vi "AG Quiz Page.vi"() -> ()   [LabVIEW 2012]
uses:
  Controls/Quiz Question.ctl
  Controls/StoredQuizAnswer.ctl
  Controls/Solution Type enum.ctl
  Controls/Problem Type enum.ctl
  Controls/Quiz Set Up.ctl
panel:
  in  "Previous 2":bool
  out "Student Answers":string[](array[string])
  in  "Resources":path[](array[path])
  in  "Previous":bool
  in  "Next":bool
  in  "Quiz Scrollbar":i32(c297)
  in  "Problem3":T1={"ProblemNum"=0, "Problem Type"={"Text"="", "Image"=bytes[0], "Text&Image"={"Text (&Image)"="", "Image (&text)"=bytes[0]}}, "Solution Type"={"Short Answer"="", "True/False"=enum."True", "Radio"=enum."E", "Multi"={"Numeric"=0.0, "String"="", "A"=FALSE, "B"=FALSE, "C"=FALSE, "D"=FALSE, "E"=TRUE}}, "Answer Color"=0, "Submit"=FALSE}
  in  "Problem2":T1={"ProblemNum"=0, "Problem Type"={"Text"="", "Image"=bytes[0], "Text&Image"={"Text (&Image)"="", "Image (&text)"=bytes[0]}}, "Solution Type"={"Short Answer"="", "True/False"=enum."True", "Radio"=enum."E", "Multi"={"Numeric"=0.0, "String"="", "A"=FALSE, "B"=FALSE, "C"=FALSE, "D"=FALSE, "E"=TRUE}}, "Answer Color"=0, "Submit"=FALSE}
  in  "Problem1":T1={"ProblemNum"=0, "Problem Type"={"Text"="", "Image"=bytes[0], "Text&Image"={"Text (&Image)"="", "Image (&text)"=bytes[0]}}, "Solution Type"={"Short Answer"="", "True/False"=enum."True", "Radio"=enum."E", "Multi"={"Numeric"=0.0, "String"="", "A"=FALSE, "B"=FALSE, "C"=FALSE, "D"=FALSE, "E"=TRUE}}, "Answer Color"=0, "Submit"=FALSE}
  in  "Problem0":T1={"ProblemNum"=0, "Problem Type"={"Text"="", "Image"=bytes[0], "Text&Image"={"Text (&Image)"="", "Image (&text)"=bytes[0]}}, "Solution Type"={"Short Answer"="", "True/False"=enum."True", "Radio"=enum."E", "Multi"={"Numeric"=0.0, "String"="", "A"=FALSE, "B"=FALSE, "C"=FALSE, "D"=FALSE, "E"=TRUE}}, "Answer Color"=0, "Submit"=FALSE}
  out "Quiz Set up Array":T2[](array[typedef])=[{"Text"="", "Problem Type"=enum."Text", "Solution Type"=enum."Text", "NumSolMin"=0.0, "NumSolMax"=0.0, "NumSolSigFig"=0, "StoreAnswer"=variant, "Picture"=bytes[0], "T/F_Solution"=FALSE, "ExactMatch"=FALSE, "TextAnswer"="", "MultiAnswer"={"MultiDescArray"=[], "MultiBoolArray"=[]}, "SigFig?"=FALSE}, {"Text"="", "Problem Type"=enum."Text", "Solution Type"=enum."Text", "NumSolMin"=0.0, "NumSolMax"=0.0, "NumSolSigFig"=0, "StoreAnswer"=variant, "Picture"=bytes[0], "T/F_Solution"=FALSE, "ExactMatch"=FALSE, "TextAnswer"="", "MultiAnswer"={"MultiDescArray"=[], "MultiBoolArray"=[]}, "SigFig?"=FALSE}, {"Text"="", "Problem Type"=enum."Text", "Solution Type"=enum."Text", "NumSolMin"=0.0, "NumSolMax"=0.0, "NumSolSigFig"=0, "StoreAnswer"=variant, "Picture"=bytes[0], "T/F_Solution"=FALSE, "ExactMatch"=FALSE, "TextAnswer"="", "MultiAnswer"={"MultiDescArray"=[], "MultiBoolArray"=[]}, "SigFig?"=FALSE}, {"Text"="", "Problem Type"=enum."Text", "Solution Type"=enum."Text", "NumSolMin"=0.0, "NumSolMax"=0.0, "NumSolSigFig"=0, "StoreAnswer"=variant, "Picture"=bytes[0], "T/F_Solution"=FALSE, "ExactMatch"=FALSE, "TextAnswer"="", "MultiAnswer"={"MultiDescArray"=[], "MultiBoolArray"=[]}, "SigFig?"=FALSE}]
  in  "stop":bool
  # "C:\\Users\\NIK12\\Desktop\\AG Quiz Image - Art.png"
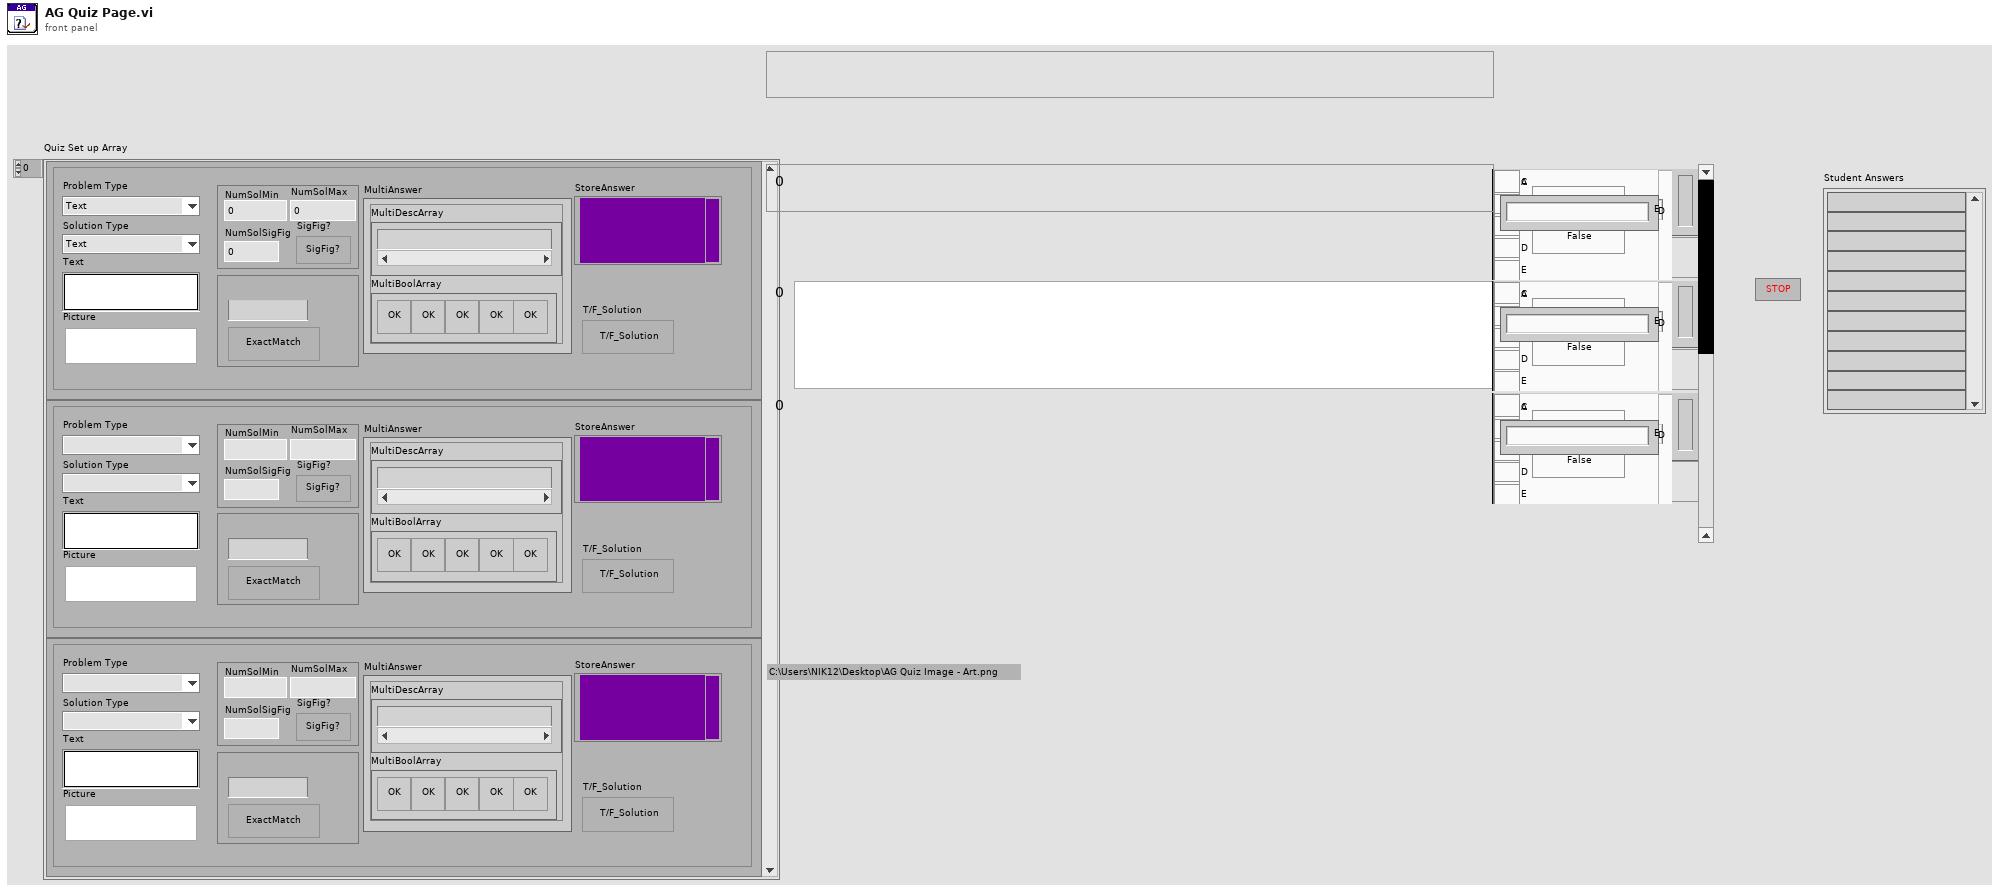
[diagram p1: front panel]
types:
  T1 = typedef "Quiz Question.ctl" = cluster{"ProblemNum":i32, "Problem Type":cluster{"Text":string, "Image":picture, "Text&Image":cluster{"Text (&Image)":string, "Image (&text)":picture}}, "Solution Type":cluster{"Short Answer":string, "True/False":enum32{"No Selection", "True", "False"}, "Radio":enum32{"E", "D", "C", "B", "A"}, "Multi":cluster{"Numeric":dbl, "String":string, "A":bool, "B":bool, "C":bool, "D":bool, "E":bool}}, "Answer Color":u32, "Submit":bool}
  T2 = typedef "Quiz Set Up.ctl" = cluster{"Text":string, "Problem Type":T3, "Solution Type":T4, "NumSolMin":dbl, "NumSolMax":dbl, "NumSolSigFig":u32, "StoreAnswer":variant, "Picture":picture, "T/F_Solution":bool, "ExactMatch":bool, "TextAnswer":string, "MultiAnswer":cluster{"MultiDescArray":string[], "MultiBoolArray":bool[]}, "SigFig?":bool}
  T3 = typedef "Problem Type enum.ctl" = enum16{"Text", "Image", "Text&Image"}
  T4 = typedef "Solution Type enum.ctl" = enum16{"Numeric", "Text", "SelectMultiple", "SelectOne", "True/False", "ShortAnswer"}
  T5 = typedef "StoredQuizAnswer.ctl" = cluster{"Solution Type":cluster{"NumAnswer":dbl, "StringAnswer":string, "MultiAnswer":cluster{"MultiAnswer":bool[], "MultiText":string[]}, "RadioAnswer":enum32{"No Selection", "Radio Selection 5", "Radio Selection 6", "Radio Selection 7", "Radio Selection 8", "Radio Selection 9"}, "TrueFalseAnswer":enum32{"No Selection", "True", "False"}, "ShortAnswer":string}, "Answer State":enum16{"Unanswered", "Correct", "Incorrect"}}
  T6 = cluster{"Short Answer":string, "True/False":enum32{"No Selection", "True", "False"}, "Radio":enum32{"E", "D", "C", "B", "A"}, "Multi":cluster{"Numeric":dbl, "String":string, "A":bool, "B":bool, "C":bool, "D":bool, "E":bool}}
  T7 = cluster{"MultiDescArray":string[], "MultiBoolArray":bool[]}
  T8 = cluster{"Numeric":dbl, "String":string, "A":bool, "B":bool, "C":bool, "D":bool, "E":bool}
  T9 = cluster{"Numeric":dbl, "String":dbl, "A":dbl, "B":dbl, "C":dbl, "D":dbl, "E":dbl}
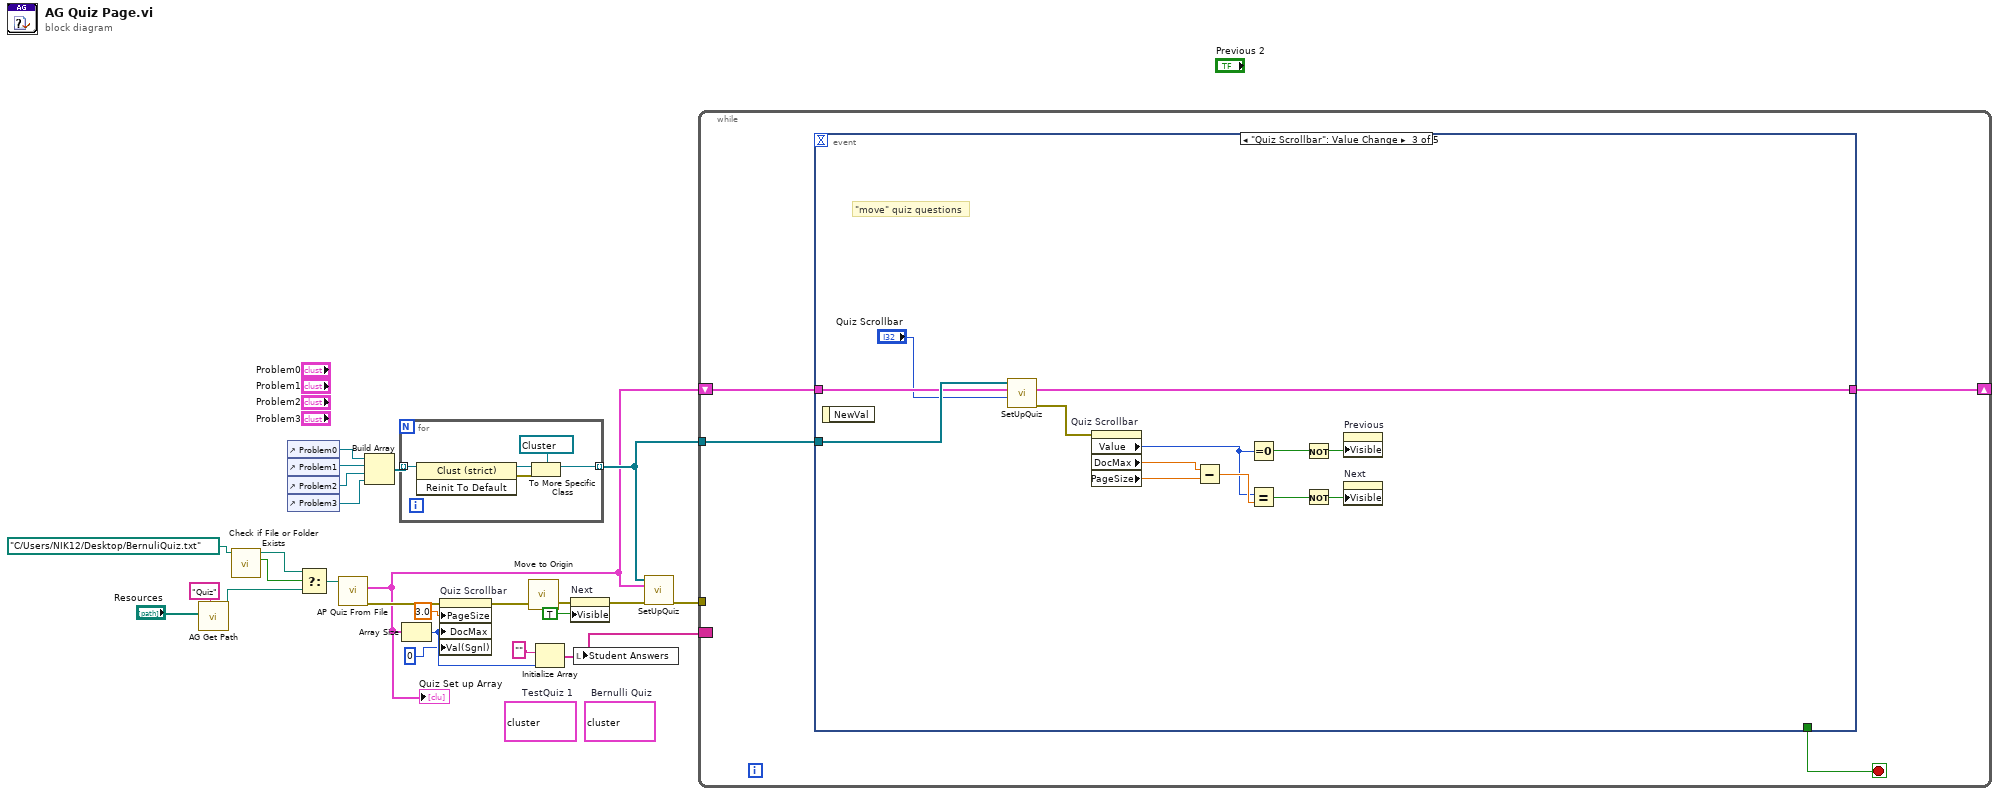
[diagram p0: block diagram]
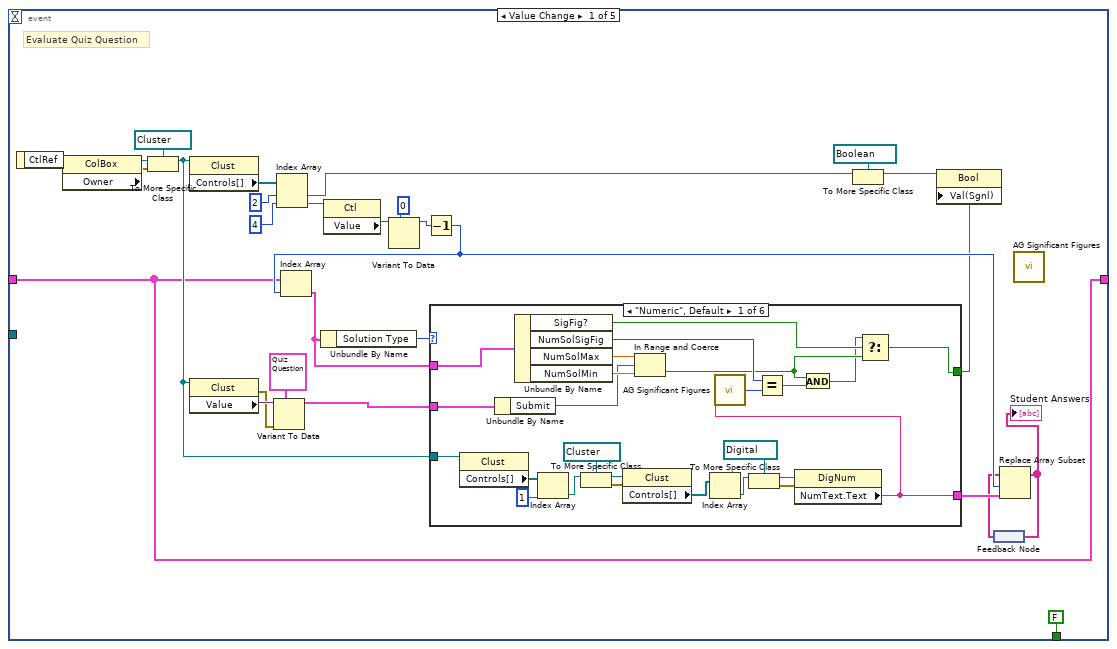
[diagram p2: hidden frame]
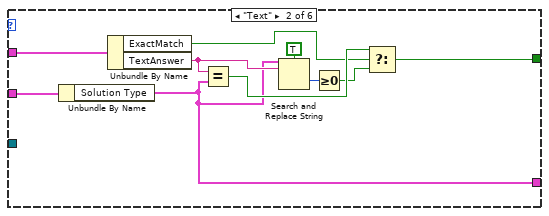
[diagram p3: hidden frame]
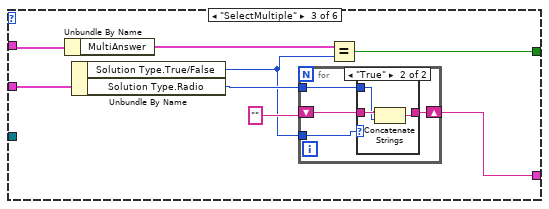
[diagram p4: hidden frame]
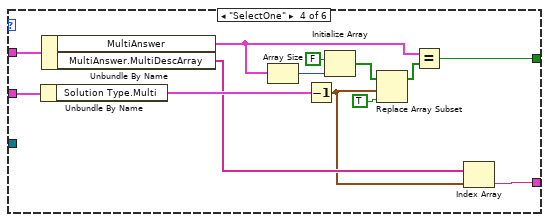
[diagram p6: hidden frame]
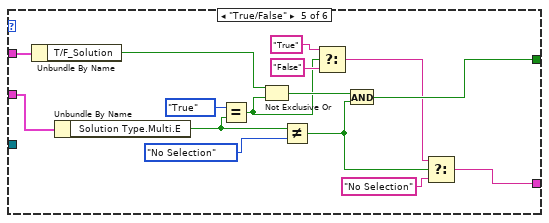
[diagram p7: hidden frame]
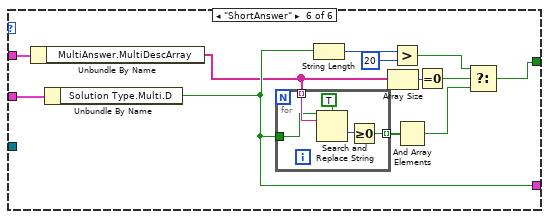
[diagram p8: hidden frame]
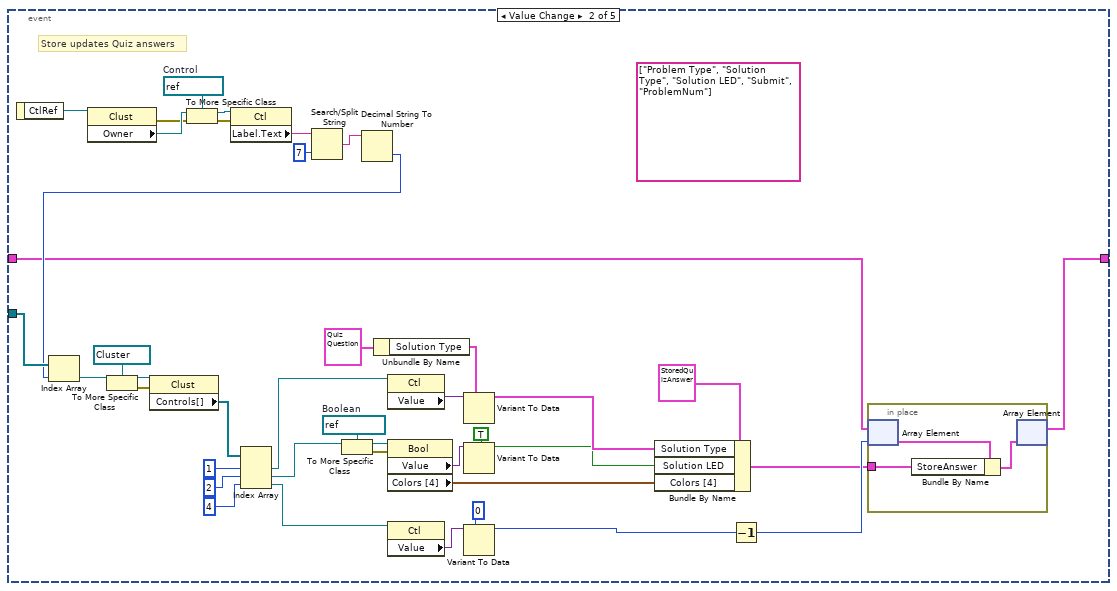
[diagram p9: hidden frame]
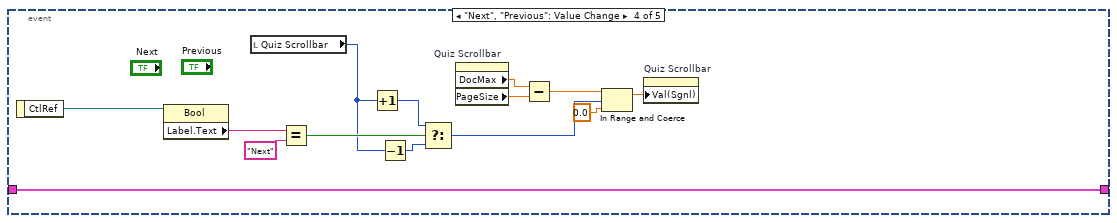
[diagram p10: hidden frame]
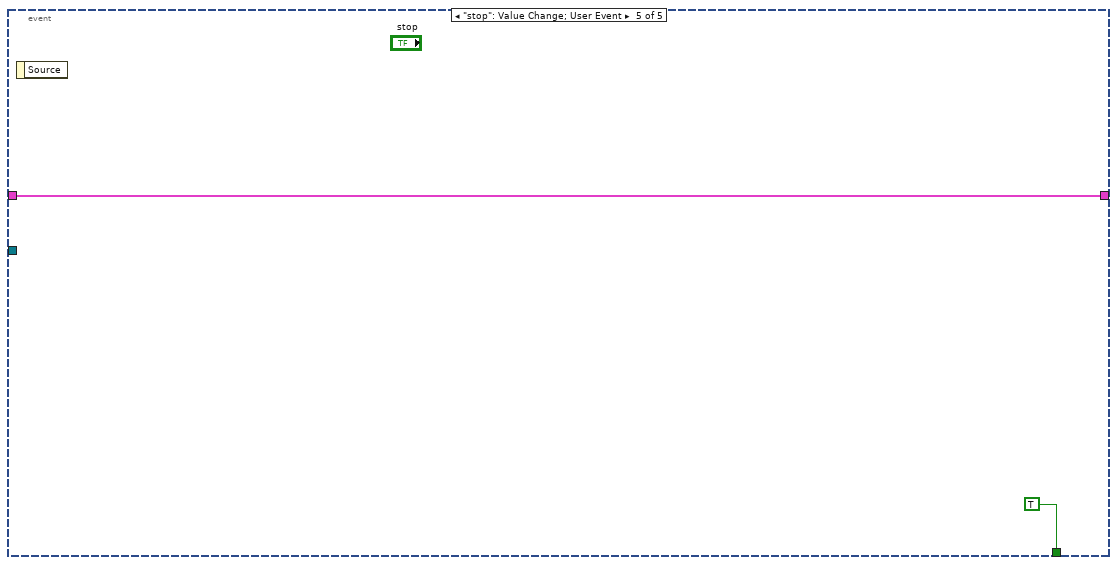
[diagram p11: hidden frame]
diagram:
  (unwired) T2[] [{"Text"="", "Problem Type"=enum."Text", "Solution Type"=enum."Numeric", "NumSolMin"=0.0, "NumSolMax"=0.0, "NumSolSigFig"=0, "StoreAnswer"=variant, "Picture"=bytes[0], "T/F_Solution"=FALSE, "ExactMatch"=FALSE, "TextAnswer"="", "MultiAnswer"={"MultiDescArray"=[], "MultiBoolArray"=[]}, "SigFig?"=FALSE}, {"Text"="", "Problem Type"=enum."Text", "Solution Type"=enum."Numeric", "NumSolMin"=0.0, "NumSolMax"=0.0, "NumSolSigFig"=0, "StoreAnswer"=variant, "Picture"=bytes[0], "T/F_Solution"=FALSE, "ExactMatch"=FALSE, "TextAnswer"="", "MultiAnswer"={"MultiDescArray"=[], "MultiBoolArray"=[]}, "SigFig?"=FALSE}, {"Text"="", "Problem Type"=enum."Text", "Solution Type"=enum."Numeric", "NumSolMin"=0.0, "NumSolMax"=0.0, "NumSolSigFig"=0, "StoreAnswer"=variant, "Picture"=bytes[0], "T/F_Solution"=FALSE, "ExactMatch"=FALSE, "TextAnswer"="", "MultiAnswer"={"MultiDescArray"=[], "MultiBoolArray"=[]}, "SigFig?"=FALSE}, {"Text"="", "Problem Type"=enum."Text", "Solution Type"=enum."Numeric", "NumSolMin"=0.0, "NumSolMax"=0.0, "NumSolSigFig"=0, "StoreAnswer"=variant, "Picture"=bytes[0], "T/F_Solution"=FALSE, "ExactMatch"=FALSE, "TextAnswer"="", "MultiAnswer"={"MultiDescArray"=[], "MultiBoolArray"=[]}, "SigFig?"=FALSE}]  # Bernulli Quiz
  (unwired) T2[] [{"Text"="", "Problem Type"=enum."Text", "Solution Type"=enum."Numeric", "NumSolMin"=0.0, "NumSolMax"=0.0, "NumSolSigFig"=0, "StoreAnswer"=variant, "Picture"=bytes[0], "T/F_Solution"=FALSE, "ExactMatch"=FALSE, "TextAnswer"="", "MultiAnswer"={"MultiDescArray"=[], "MultiBoolArray"=[]}, "SigFig?"=FALSE}, {"Text"="", "Problem Type"=enum."Text", "Solution Type"=enum."Numeric", "NumSolMin"=0.0, "NumSolMax"=0.0, "NumSolSigFig"=0, "StoreAnswer"=variant, "Picture"=bytes[0], "T/F_Solution"=FALSE, "ExactMatch"=FALSE, "TextAnswer"="", "MultiAnswer"={"MultiDescArray"=[], "MultiBoolArray"=[]}, "SigFig?"=FALSE}, {"Text"="", "Problem Type"=enum."Text", "Solution Type"=enum."Numeric", "NumSolMin"=0.0, "NumSolMax"=0.0, "NumSolSigFig"=0, "StoreAnswer"=variant, "Picture"=bytes[0], "T/F_Solution"=FALSE, "ExactMatch"=FALSE, "TextAnswer"="", "MultiAnswer"={"MultiDescArray"=[], "MultiBoolArray"=[]}, "SigFig?"=FALSE}, {"Text"="", "Problem Type"=enum."Text", "Solution Type"=enum."Numeric", "NumSolMin"=0.0, "NumSolMax"=0.0, "NumSolSigFig"=0, "StoreAnswer"=variant, "Picture"=bytes[0], "T/F_Solution"=FALSE, "ExactMatch"=FALSE, "TextAnswer"="", "MultiAnswer"={"MultiDescArray"=[], "MultiBoolArray"=[]}, "SigFig?"=FALSE}, {"Text"="", "Problem Type"=enum."Text", "Solution Type"=enum."Numeric", "NumSolMin"=0.0, "NumSolMax"=0.0, "NumSolSigFig"=0, "StoreAnswer"=variant, "Picture"=bytes[0], "T/F_Solution"=FALSE, "ExactMatch"=FALSE, "TextAnswer"="", "MultiAnswer"={"MultiDescArray"=[], "MultiBoolArray"=[]}, "SigFig?"=FALSE}, {"Text"="", "Problem Type"=enum."Text", "Solution Type"=enum."Numeric", "NumSolMin"=0.0, "NumSolMax"=0.0, "NumSolSigFig"=0, "StoreAnswer"=variant, "Picture"=bytes[0], "T/F_Solution"=FALSE, "ExactMatch"=FALSE, "TextAnswer"="", "MultiAnswer"={"MultiDescArray"=[], "MultiBoolArray"=[]}, "SigFig?"=FALSE}]  # TestQuiz 1
  n1 = call "AG Get Path.vi"("Partial File Name"="Quiz", "Resources"="Resources") -> ("Path"=w3:path)  [unwired: 6 in, 3 out]
  n2 = call <vilib>:"Check if File or Folder Exists.vi"("path"=path "C:/Users/NIK12/Desktop/BernuliQuiz.txt" ("file path (dialog if empty)")) -> ("file or folder exists?"=w6:bool, "dup path"=w5:path)  [unwired: 8 in, 1 out]
  n3 = control-ref of="Problem0"() -> (w25:refnum<vi>)
  n4 = control-ref of="Problem1"() -> (w24:refnum<vi>)
  n5 = control-ref of="Problem2"() -> (w23:refnum<vi>)
  n6 = control-ref of="Problem3"() -> (w22:refnum<vi>)
  n7 = Select(t=w5, s=w6, f=w3) -> (s? t:f=w4:path)
  n8 = call "AP Quiz From File.vi"("file path (dialog if empty)"=w4) -> ("Error Out"=w10:errorcluster, "Question Array Out"=w1:T2[])  [unwired: 8 in, 1 out]
  "Quiz Set up Array" <- w1
  n9 = Build Array(w25, w24, w23, w22) -> (w21:refnum<vi>[])
  n10 = for {
    tunnel: w21 -> [w30] mode=indexing
    tunnel: [w26] -> w13 mode=indexing
    n11 = invoke class="Clust (strict)" method="Reinit To Default"(reference=w30) -> (reference out=w27:refnum<vi>, error out=w28:errorcluster)  [unwired: 2 in, 1 out]
    n12 = To More Specific Class(target class=refnum<vi> refnum ("Problem"), reference=w27, error in=w28) -> (specific class reference=w26:refnum<vi>)  [unwired: 1 out]
  }
  n13 = Array Size(array=w1) -> (size(s)=w12:i32)
  n14 = property on="Quiz Scrollbar" class="Scroll (strict)"(error in=w10, "PageSize"=3.0 ("Page Size"), "DocMax"=w12, "Val(Sgnl)"=0 ("Value (Signaling)")) -> (error out=w16:errorcluster)  [unwired: 1 in, 1 out]
  n15 = call "Move to Origin.vi"("Error In"=w16) -> ("Error Out"=w17:errorcluster)  [unwired: 2 in]
  n16 = Initialize Array("" ("Answer Array"), w12) -> (w18:string[])
  n17 = property on="Next" class="Bool"(error in=w17, "Visible"=TRUE) -> (error out=w15:errorcluster)  [unwired: 1 in, 1 out]
  n18 = local write "Student Answers"(w18) -> ()
  n19 = call "SetUpQuiz.vi"("Error In"=w15, "Quiz Set Up info"=w1, "? Ref Array"=w13) -> ("Error Out"=w14:errorcluster)  [unwired: 7 in, 1 out]
  n20 = while {
    tunnel: w13 -> [w31]
    border: w18 -> [_]
    tunnel: w14 -> [_]
    shift-right: [w32] -> _
    shift-left: w1 -> [w33]
    stop <- w34 stop-if-true
    n21 = event shown="[2] \"Quiz Scrollbar\": Value Change" {
      selector: _ -> [_ _ _ _ _]
      dyn-events: _ -> [_ _ _ _ _]
      timeout: _ -> [_ _ _ _ _]
      tunnel: w31 -> [_ w191 w207 _ _]
      tunnel: [FALSE _ _ _ TRUE] -> w34
      tunnel: w33 -> [w39 w179 w205 w217 w230]
      tunnel: [w39 w178 w204 w217 w230] -> w32
      event Value Change {
        # "Evaluate Quiz Question"
        n22 = event-data() -> ("CtlRef"=w37:refnum<vi>)  [unwired: 1 in]
        n23 = property on="Property Node" class="ColBox"(reference=w37) -> (error out=w40:errorcluster, "Owner"=w59:refnum<vi>)  [unwired: 1 in, 1 out]
        n24 = To More Specific Class(target class=refnum<vi> refnum ("Problem"), reference=w59, error in=w40) -> (specific class reference=w41:refnum<vi>)  [unwired: 1 out]
        n25 = property on="Property Node" class="Clust"(reference=w41) -> ("Controls[]"=w56:refnum<vi>[])  [unwired: 1 in, 2 out]
        n26 = property on="Property Node" class="Clust"(reference=w41) -> (error out=w36:errorcluster, "Value"=w51:variant)  [unwired: 1 in, 1 out]
        n27 = Variant To Data(error in=w36, type=T1 {"ProblemNum"=0, "Problem Type"={"Text"="", "Image"=bytes[0], "Text&Image"={"Text (&Image)"="", "Image (&text)"=bytes[0]}}, "Solution Type"={"Short Answer"="", "True/False"=enum."No Selection", "Radio"=enum."E", "Multi"={"Numeric"=0.0, "String"="", "A"=FALSE, "B"=FALSE, "C"=FALSE, "D"=FALSE, "E"=FALSE}}, "Answer Color"=0, "Submit"=FALSE} ("Problem"), Variant=w51) -> (data=w49:T1)  [unwired: 1 out]
        n28 = Index Array(array=w56, index #1=2 ("index"), index #2=4 ("index")) -> (element #1=w38:refnum<vi>, element #2=w45:refnum<vi>)
        n29 = property on="Property Node" class="Ctl"(reference=w45) -> ("Value"=w44:variant)  [unwired: 1 in, 2 out]
        n30 = Variant To Data(type=0, Variant=w44) -> (data=w42:i32)  [unwired: 1 in, 1 out]
        n31 = Decrement(x=w42) -> (x-1=w61:i32)
        n32 = Index Array(array=w39, index=w61) -> (element=w47:T2)
        n33 = Unbundle By Name(w47) -> ("Solution Type"=w57:T4)
        n34 = case shown="\"Numeric\", Default" w57 {
          tunnel: w47 -> [w87 w97 w104 w126 w140 w143]
          tunnel: [w66 w91 w102 w124 w134 w144] -> w52
          tunnel: w49 -> [w84 w96 w105 w125 w141 w153]
          tunnel: [w70 w89 w100 w116 w127 w150] -> w62
          tunnel: w41 -> [w82 _ _ _ _ _]
          frame "Numeric", Default {
            n35 = property on="Property Node" class="Clust"(reference=w82) -> ("Controls[]"=w81:refnum<vi>[])  [unwired: 1 in, 2 out]
            n36 = Unbundle By Name(w84) -> ("Submit"=w83:bool)
            n37 = Unbundle By Name(w87) -> ("SigFig?"=w67:bool, "NumSolSigFig"=w69:u32, "NumSolMax"=w85:dbl, "NumSolMin"=w86:dbl)
            n38 = Index Array(array=w81, index=1) -> (element=w79:refnum<vi>)
            n39 = To More Specific Class(target class=refnum<vi> refnum ("Problem Type"), reference=w79) -> (specific class reference=w76:refnum<vi>, error out=w77:errorcluster)  [unwired: 1 in]
            n40 = property on="Property Node" class="Clust"(reference=w76, error in=w77) -> ("Controls[]"=w75:refnum<vi>[])  [unwired: 2 out]
            n41 = In Range and Coerce(upper limit=w85, x=w83, lower limit=w86) -> (In Range?=w64:bool)  [unwired: 1 out]
            n42 = Index Array(array=w75) -> (element=w74:refnum<vi>)  [unwired: 1 in]
            n43 = To More Specific Class(target class=refnum<vi> refnum ("Problem Type"), reference=w74) -> (specific class reference=w72:refnum<vi>, error out=w71:errorcluster)  [unwired: 1 in]
            n44 = property on="Property Node" class="DigNum"(reference=w72, error in=w71) -> ("NumText.Text"=w70:string)  [unwired: 2 out]
            n45 = call "AG Significant Figures.vi"("String Number"=w70) -> ("Significant Figures"=w68:i32)  [unwired: 13 in, 1 out]
            n46 = Equal?(x=w69, y=w68) -> (x = y?=w65:bool)
            n47 = And(x=w64, y=w65) -> (x .and. y?=w63:bool)
            n48 = Select(t=w63, s=w67, f=w64) -> (s? t:f=w66:bool)
          }
          frame "Text" {
            n49 = Unbundle By Name(w96) -> ("Solution Type"=w89:T6)
            n50 = Unbundle By Name(w97) -> ("ExactMatch"=w88:bool, "TextAnswer"=w90:string)
            n51 = Equal?(x=w90, y=w89) -> (x = y?=w93:bool)
            n52 = Search and Replace String(case sensitive?=TRUE ("ignore case? (F)"), input string=w89, search string=w90) -> (offset past replacement=w94:i32)  [unwired: 5 in, 3 out]
            n53 = Greater Or Equal To 0?(x=w94) -> (x >= 0?=w92:bool)
            n54 = Select(t=w93, s=w88, f=w92) -> (s? t:f=w91:bool)
          }
          frame "SelectMultiple" {
            n55 = Unbundle By Name(w104) -> ("MultiAnswer"=w103:T7)
            n56 = Unbundle By Name(w105) -> ("Solution Type.True/False"=w98:enum32{"No Selection", "True", "False"}, "Solution Type.Radio"=w99:enum32{"E", "D", "C", "B", "A"})
            n57 = for {
              shift-right: [w108] -> w100
              shift-left: "" -> [w109]
              tunnel: w99 -> [w107]
              tunnel: w98 -> [w106]
              n58 = case shown="\"True\"" w106 {
                tunnel: w109 -> [w110 w113]
                tunnel: [w110 w112] -> w108
                tunnel: w107 -> [_ w111]
                frame "No Selection", Default {
                }
                frame "True" {
                  n59 = Concatenate Strings(w113, w111) -> (w112:string)
                }
              }
            }
            n60 = Equal?(x=w103, y=w98) -> (x = y?=w102:bool)
          }
          frame "SelectOne" {
            n61 = Unbundle By Name(w125) -> ("Solution Type.Multi"=w121:T8)
            n62 = Unbundle By Name(w126) -> ("MultiAnswer"=w114:T7, "MultiAnswer.MultiDescArray"=w118:string[])
            n63 = Array Size(array=w114) -> (size(s)=w122:i32)
            n64 = Decrement(x=w121) -> (x-1=w117:T9)
            n65 = Initialize Array(FALSE, w122) -> (w120:bool[])
            n66 = Replace Array Subset(array=w120, new element=TRUE ("new element/subarray"), index=w117) -> (w115:bool[])
            n67 = Equal?(x=w114, y=w115) -> (x = y?=w124:bool)
            n68 = Index Array(array=w118, index=w117) -> (element=w116:string)
          }
          frame "True/False" {
            n69 = Unbundle By Name(w140) -> ("T/F_Solution"=w139:bool)
            n70 = Unbundle By Name(w141) -> ("Solution Type.Multi.E"=w137:bool)
            n71 = Equal?(x=enum32{"No Selection", "True", "False"}."True" ("Solution Type.TrueFalseAnswer"), y=w137) -> (x = y?=w129:bool)
            n72 = Not Exclusive Or(1:w129, 2:w139) -> (0:w135:bool)
            n73 = Not Equal?(x=w137, y=enum32{"No Selection", "True", "False"}."No Selection" ("Solution Type.TrueFalseAnswer")) -> (x != y?=w133:bool)
            n74 = Select(t="True", s=w129, f="False") -> (s? t:f=w128:string)
            n75 = And(x=w135, y=w133) -> (x .and. y?=w134:bool)
            n76 = Select(t=w128, s=w133, f="No Selection") -> (s? t:f=w127:string)
          }
          frame "ShortAnswer" {
            n77 = Unbundle By Name(w143) -> ("MultiAnswer.MultiDescArray"=w142:string[])
            n78 = Unbundle By Name(w153) -> ("Solution Type.Multi.D"=w150:bool)
            n79 = for {
              tunnel: w150 -> [w156]
              tunnel: w142 -> [w157] mode=indexing
              tunnel: [w158] -> w149 mode=indexing
              n80 = Search and Replace String(case sensitive?=TRUE ("ignore case? (F)"), input string=w156, search string=w157) -> (offset past replacement=w155:i32)  [unwired: 5 in, 3 out]
              n81 = Greater Or Equal To 0?(x=w155) -> (x >= 0?=w158:bool)
            }
            n82 = String Length(string=w150) -> (length=w152:i32)
            n83 = Array Size(array=w142) -> (size(s)=w148:i32)
            n84 = Greater?(x=w152, y=20 ("x")) -> (0:w146:bool)
            n85 = And Array Elements(Boolean array=w149) -> (logical AND=w145:bool)
            n86 = Equal To 0?(x=w148) -> (x = 0?=w147:bool)
            n87 = Select(t=w146, s=w147, f=w145) -> (s? t:f=w144:bool)
          }
        }
        n88 = To More Specific Class(target class=refnum<vi> refnum ("SigFig?"), reference=w38) -> (specific class reference=w53:refnum<vi>)  [unwired: 1 in, 1 out]
        n89 = property on="Property Node" class="Bool"(reference=w53, "Val(Sgnl)"=w52) -> ()  [unwired: 1 in, 2 out]
        n90 = feedback #1() -> (w58:string[])
        n91 = Replace Array Subset(array=w58, new element=w62, index=w61) -> (w35:string[])
        "Student Answers" <- w35
        n92 = feedback-in #1(w35) -> ()
        n93 = call "AG Significant Figures.vi"() -> ()  [unwired: 14 in, 2 out]
      }
      event Value Change {
        (unwired) string[] ["Problem Type", "Solution Type", "Solution LED", "Submit", "ProblemNum"] ("Array")
        w174 = refnum<vi> refnum  # Boolean
        w194 = refnum<vi> refnum  # Control
        # "Store updates Quiz answers"
        n94 = event-data() -> ("CtlRef"=w199:refnum<vi>)  [unwired: 1 in]
        n95 = property on="Property Node" class="Clust"(reference=w199) -> (error out=w195:errorcluster, "Owner"=w198:refnum<vi>)  [unwired: 1 in, 1 out]
        n96 = To More Specific Class(target class=w194, reference=w198, error in=w195) -> (specific class reference=w197:refnum<vi>, error out=w196:errorcluster)
        n97 = property class="Ctl"(reference=w197, error in=w196) -> ("Label.Text"=w193:string)  [unwired: 2 out]
        n98 = Search/Split String(string=w193, offset (0)=7) -> (match + rest of string=w190:string)  [unwired: 1 in, 2 out]
        n99 = Decimal String To Number(string=w190) -> (number=w189:i32)  [unwired: 2 in, 1 out]
        n100 = Index Array(array=w191, index=w189) -> (element=w187:refnum<vi>)
        n101 = To More Specific Class(target class=refnum<vi> refnum ("Problem"), reference=w187) -> (specific class reference=w186:refnum<vi>, error out=w185:errorcluster)  [unwired: 1 in]
        n102 = property on="Property Node" class="Clust"(reference=w186, error in=w185) -> ("Controls[]"=w160:refnum<vi>[])  [unwired: 2 out]
        n103 = Index Array(array=w160, index #1=1 ("index"), index #2=2 ("index"), index #3=4 ("index")) -> (element #1=w166:refnum<vi>, element #2=w176:refnum<vi>, element #3=w161:refnum<vi>)
        n104 = To More Specific Class(target class=w174, reference=w176) -> (specific class reference=w175:refnum<vi>, error out=w165:errorcluster)  [unwired: 1 in]
        n105 = Unbundle By Name(T1 {"ProblemNum"=0, "Problem Type"={"Text"="", "Image"=bytes[0], "Text&Image"={"Text (&Image)"="", "Image (&text)"=bytes[0]}}, "Solution Type"={"Short Answer"="", "True/False"=enum."No Selection", "Radio"=enum."E", "Multi"={"Numeric"=0.0, "String"="", "A"=FALSE, "B"=FALSE, "C"=FALSE, "D"=FALSE, "E"=FALSE}}, "Answer Color"=0, "Submit"=FALSE} ("Problem")) -> ("Solution Type"=w170:T6)
        n106 = property on="Property Node" class="Ctl"(reference=w166) -> ("Value"=w172:variant)  [unwired: 1 in, 2 out]
        n107 = property on="Property Node" class="Bool"(reference=w175, error in=w165) -> ("Value"=w168:variant, "Colors [4]"=w163:cluster{u32, u32}[])  [unwired: 2 out]
        n108 = property on="Property Node" class="Ctl"(reference=w161) -> ("Value"=w183:variant)  [unwired: 1 in, 2 out]
        n109 = Variant To Data(type=w170, Variant=w172) -> (data=w171:T6)  [unwired: 1 in, 1 out]
        n110 = Variant To Data(type=TRUE, Variant=w168) -> (data=w169:bool)  [unwired: 1 in, 1 out]
        n111 = Variant To Data(type=0, Variant=w183) -> (data=w181:i32)  [unwired: 1 in, 1 out]
        n112 = Bundle By Name(cluster=T5 {"Solution Type"={"NumAnswer"=0.0, "StringAnswer"="", "MultiAnswer"={"MultiAnswer"=[], "MultiText"=[]}, "RadioAnswer"=enum."No Selection", "TrueFalseAnswer"=enum."No Selection", "ShortAnswer"=""}, "Answer State"=enum."Unanswered"} ("output cluster"), "Solution Type"=w171, "Solution LED"=w169, "Colors [4]"=w163) -> (w167:T5)
        n113 = Decrement(x=w181) -> (x-1=w180:i32)
        n114 = in-place {
          in-place-border: w167 -> [w200]
          n115 = in-place-array #2(w179, w180) -> (w202:T2)
          n116 = Bundle By Name(cluster=w202, "StoreAnswer"=w200) -> (w201:T2)
          n117 = in-place-array #2(w201) -> (w178:T2[])  [unwired: 1 out]
        }
      }
      event "Quiz Scrollbar": Value Change {
        # "\"move\" quiz questions"
        n118 = event-data() -> ()  [unwired: 1 in, 1 out]
        n119 = call "SetUpQuiz.vi"("Problem Offset (0)"="Quiz Scrollbar", "Quiz Set Up info"=w205, "? Ref Array"=w207) -> ("Error Out"=w206:errorcluster, "Quiz Set Up Out"=w204:T2[])  [unwired: 7 in]
        n120 = property on="Quiz Scrollbar" class="Scroll (strict)"(error in=w206) -> ("Value"=w210:i32, "DocMax"=w215:dbl, "PageSize"=w214:dbl)  [unwired: 1 in, 2 out]
        n121 = Subtract(x=w215, y=w214) -> (x-y=w213:dbl)
        n122 = Equal To 0?(x=w210) -> (x = 0?=w208:bool)
        n123 = Equal?(x=w210, y=w213) -> (x = y?=w211:bool)
        n124 = Not(x=w208) -> (.not. x?=w209:bool)
        n125 = Not(x=w211) -> (.not. x?=w212:bool)
        n126 = property on="Previous" class="Bool"("Visible"=w209) -> ()  [unwired: 2 in, 2 out]
        n127 = property on="Next" class="Bool"("Visible"=w212) -> ()  [unwired: 2 in, 2 out]
      }
      event "Next", "Previous": Value Change {
        n128 = event-data() -> ("CtlRef"=w222:refnum<vi>)  [unwired: 1 in]
        n129 = property class="Bool"(reference=w222) -> ("Label.Text"=w221:string)  [unwired: 1 in, 2 out]
        n130 = local read "Quiz Scrollbar"() -> (w216:i32)
        n131 = Equal?(x=w221, y="Next") -> (x = y?=w219:bool)
        n132 = Increment(x=w216) -> (x+1=w224:i32)
        n133 = Decrement(x=w216) -> (x-1=w223:i32)
        n134 = Select(t=w224, s=w219, f=w223) -> (s? t:f=w218:i32)
        n135 = property on="Quiz Scrollbar" class="Scroll (strict)"() -> ("DocMax"=w229:dbl, "PageSize"=w225:dbl)  [unwired: 2 in, 2 out]
        n136 = Subtract(x=w229, y=w225) -> (x-y=w226:dbl)
        n137 = In Range and Coerce(upper limit=w226, x=w218, lower limit=0.0) -> (coerced(x)=w228:dbl)  [unwired: 1 out]
        n138 = property on="Quiz Scrollbar" class="Scroll (strict)"("Val(Sgnl)"=w228) -> ()  [unwired: 2 in, 2 out]
      }
      event "stop": Value Change; User Event {
        n139 = event-data() -> ()  [unwired: 1 in, 1 out]
      }
    }
  }
